vi "Result Set Data.vi"(8 "error in":errorcluster, 9 "Set Data":T1={"UUT_TEST_INFO"={"ID"="", "STATION_ID"="", "TEST_SOCKET_INDEX"="", "UUT_SERIAL_NUMBER"="", "TSW_VER"="", "VAL_SW_VER"="", "PROJECT_NAME"="", "PRODUCT_NAME"="", "PRODUCT_VARIANT"="", "TEST_NAME"="", "TEST_PHASE"="", "TEST_DESCRIPTION"="", "TEMP_CHAMBER_NAME"="", "START_DATE_TIME"="", "STOP_DATE_TIME "="", "START_CYCLE_COUNT"="", "STOP_CYCLE_COUNT"="", "EXECUTION_TIME"="", "UUT_STATUS"="", "UUT_ERROR_CODE"="", "UUT_ERROR_MESSAGE"="", "TEST_SEQUENCE"=""}, "FE_FRAME_LOG"={"ID"="", "UUT_TEST_INFO"="", "DATE_TIME"="", "CYCLE_NUMBER"="", "TEST_MODE"="", "CHAMBER_TEMP"="", "CAN_FRAME_RX"="", "Test Mode"=0, "LV_PPS_VOLTAGE"="", "LV_PPS_CURRENT"="", "HV_PPS_VOLTAGE"="", "HV_PPS_CURRENT"="", "SOCKET_NUMBER"="", "CAN_FRAME_RX_NO_OFF_BYTE"=""}, "FF_FRAME_LOG"={"ID"="", "UUT_TEST_INFO"="", "DATE_TIME"="", "CYCLE_NUMBER"="", "TEST_MODE"="", "CAN_FRAME_RX"="", "CHAMBER_TEMP"="", "TestMode"=0, "SOCKET_NUMBER"="", "CAN_FRAME_RX_NO_OFF_BYTE"=""}, "LIMIT_TABLE"={"ID"="", "PRODUCT_NAME"="", "PRODUCT_VARIANT"="", "TEST_MODE"="", "PARAMETER_NAME"="", "COMPARISON_TYPE"="", "LOW_LIMIT"="", "HIGH_LIMIT"="", "UNIT"="", "ERROR_MESSSAGE"="", "SEVERITY"=""}, "ERROR LOG Append"=[], "FA_FRAME_LOG"={"UUT_TEST_INFO"="", "CAN_FRAME_RX"="", "CAN_FRAME_RX_NO_OFF_BYTE"=""}, "Socket No"=1, "TEST RESULT LOG Append"=[], "SYSTEM_LOG"={"ID "="", "DATE_TIME"="", "CYCLE_NUMBER"="", "TEST_MODE"="", "ERROR_MESSAGE"=""}, "Temperature log"={"TEST_MODE"="", "CYCLE_NUMBER"="", "TEMPERATURE"={"LV_PPS_TEMPERATURE"=0.0, "HV_PPS1_TEMPERATURE"=0.0, "HV_PPS2_TEMPERATURE"=0.0, "HV_PPS3_TEMPERATURE"=0.0, "HV_PPS4_TEMPERATURE"=0.0, "HV_PPS5_TEMPERATURE"=0.0, "HV_PPS6_TEMPERATURE"=0.0, "CHAMBER_TEMPERATURE"=0.0, "LOAD_U1_TEMPERATURE"=0.0, "LOAD_V1_TEMPERATURE"=0.0, "LOAD_W1_TEMPERATURE"=0.0, "LOAD_U2_TEMPERATURE"=0.0, "LOAD_V2_TEMPERATURE"=0.0, "LOAD_W2_TEMPERATURE"=0.0, "LOAD_U3_TEMPERATURE"=0.0, "LOAD_V3_TEMPERATURE"=0.0, "LOAD_W3_TEMPERATURE"=0.0}, "Temperature Inrange"={"LVPPS_Trip?"=FALSE, "HVPPS1_Trip?"=FALSE, "HVPPS2_Trip?"=FALSE, "HVPPS3_Trip?"=FALSE, "HVPPS4_Trip?"=FALSE, "HVPPS5_Trip?"=FALSE, "HVPPS6_Trip?"=FALSE, "Chamber_Trip?"=FALSE}}, "POWER_STATUS"={"TEST_MODE"="", "CYCLE_NUMBER"="", "TYPE_POWER"="", "STATE"=""}, "CYCLE_DURATION_LOG"={"CYCLE_NUMBER"=""}}, 10 "Table Name":string, 11 "Action":enum16{"Insert", "Update"}(ring)) -> (0 "error out":errorcluster)   [LabVIEW 2023, in "HardwareAbstractionLayer_LVOOP.lvlib" / "Report.lvclass"]
uses:
  Report.lvclass
  Control/All Log Details.ctl
  Control/UUT Test Info.ctl
  Control/FE FRAME LOG.ctl
  Control/FF FRAME LOG.ctl
  Control/LIMIT TABLE.ctl
  Control/ERROR LOG APPEND.ctl
  Control/ERROR LOG.ctl
  Control/FA FRAME LOG.ctl
  Control/TEST RESULT LOG APPEND.ctl
  Control/TEST RESULT LOG.ctl
  Control/SYSTEM LOG.ctl
  Control/Temperature LOG.ctl
  Control/POWER STATUS.ctl
  Control/CYCLE_DURATION_LOG.ctl
  Control/Queue FGV.ctl
  Control/Q Data.ctl
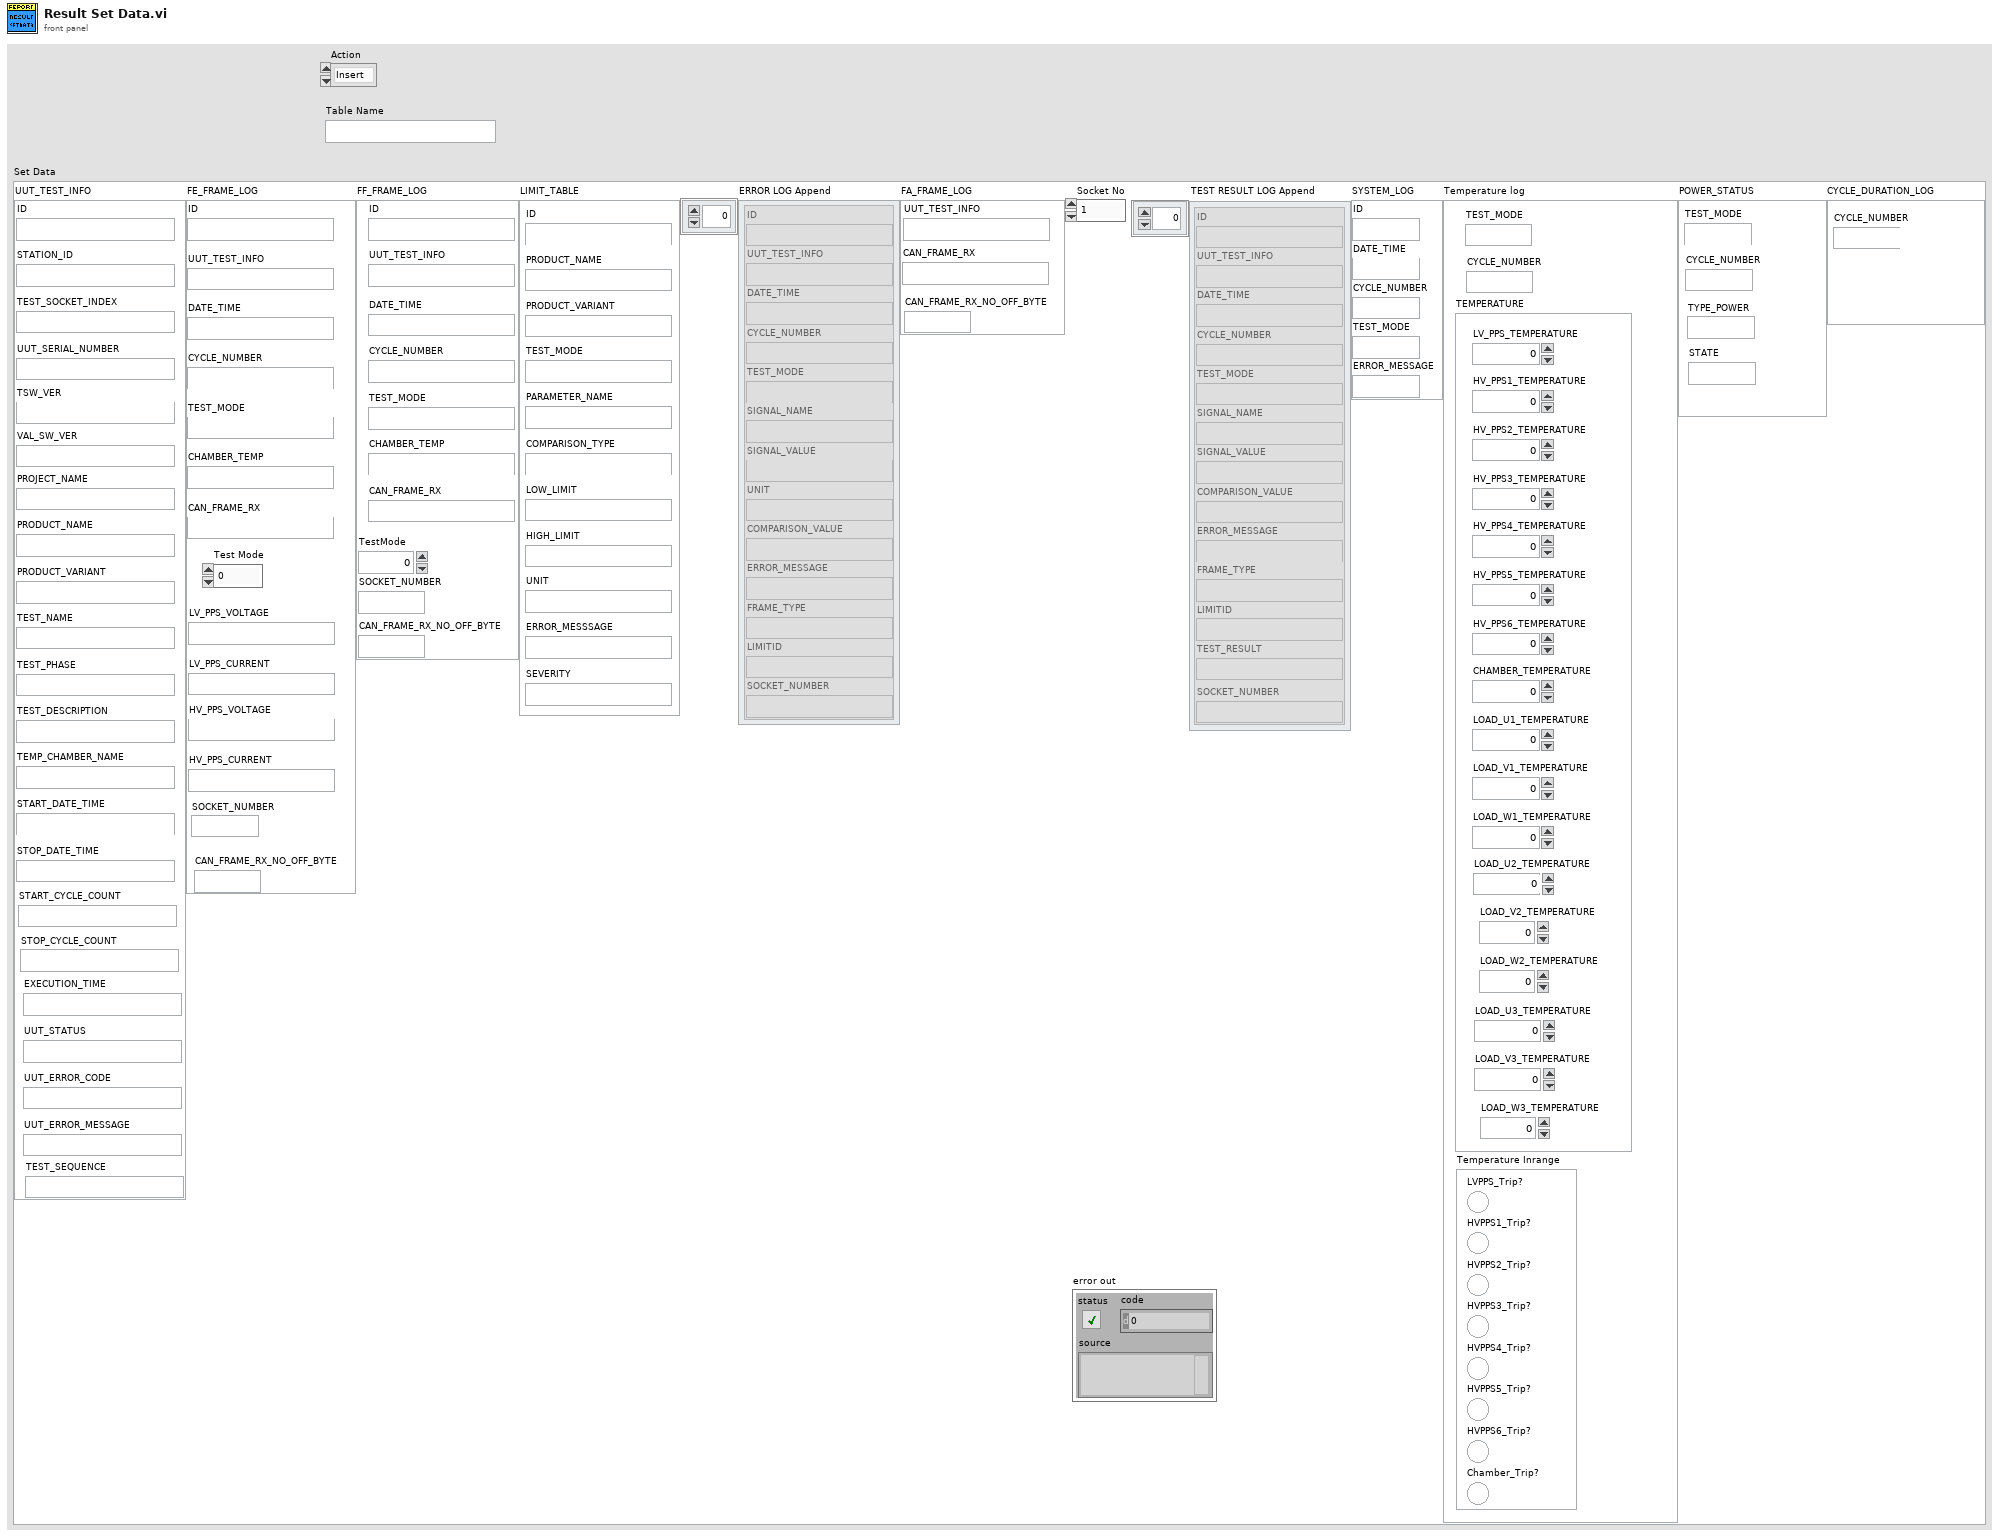
[diagram p1: front panel]
types:
  T1 = typedef "HardwareAbstractionLayer_LVOOP.lvlib/Report.lvclass/All Log Details.ctl" = cluster{"UUT_TEST_INFO":T2, "FE_FRAME_LOG":T3, "FF_FRAME_LOG":T4, "LIMIT_TABLE":T5, "ERROR LOG Append":T6, "FA_FRAME_LOG":T8, "Socket No":u16, "TEST RESULT LOG Append":T9, "SYSTEM_LOG":T11, "Temperature log":T12, "POWER_STATUS":T13, "CYCLE_DURATION_LOG":T14}
  T2 = typedef "HardwareAbstractionLayer_LVOOP.lvlib/Report.lvclass/UUT Test Info.ctl" = cluster{"ID":string, "STATION_ID":string, "TEST_SOCKET_INDEX":string, "UUT_SERIAL_NUMBER":string, "TSW_VER":string, "VAL_SW_VER":string, "PROJECT_NAME":string, "PRODUCT_NAME":string, "PRODUCT_VARIANT":string, "TEST_NAME":string, "TEST_PHASE":string, "TEST_DESCRIPTION":string, "TEMP_CHAMBER_NAME":string, "START_DATE_TIME":string, "STOP_DATE_TIME ":string, "START_CYCLE_COUNT":string, "STOP_CYCLE_COUNT":string, "EXECUTION_TIME":string, "UUT_STATUS":string, "UUT_ERROR_CODE":string, "UUT_ERROR_MESSAGE":string, "TEST_SEQUENCE":string}
  T3 = typedef "HardwareAbstractionLayer_LVOOP.lvlib/Report.lvclass/FE FRAME LOG.ctl" = cluster{"ID":string, "UUT_TEST_INFO":string, "DATE_TIME":string, "CYCLE_NUMBER":string, "TEST_MODE":string, "CHAMBER_TEMP":string, "CAN_FRAME_RX":string, "Test Mode":u32, "LV_PPS_VOLTAGE":string, "LV_PPS_CURRENT":string, "HV_PPS_VOLTAGE":string, "HV_PPS_CURRENT":string, "SOCKET_NUMBER":string, "CAN_FRAME_RX_NO_OFF_BYTE":string}
  T4 = typedef "HardwareAbstractionLayer_LVOOP.lvlib/Report.lvclass/FF FRAME LOG.ctl" = cluster{"ID":string, "UUT_TEST_INFO":string, "DATE_TIME":string, "CYCLE_NUMBER":string, "TEST_MODE":string, "CAN_FRAME_RX":string, "CHAMBER_TEMP":string, "TestMode":u32, "SOCKET_NUMBER":string, "CAN_FRAME_RX_NO_OFF_BYTE":string}
  T5 = typedef "HardwareAbstractionLayer_LVOOP.lvlib/Report.lvclass/LIMIT TABLE.ctl" = cluster{"ID":string, "PRODUCT_NAME":string, "PRODUCT_VARIANT":string, "TEST_MODE":string, "PARAMETER_NAME":string, "COMPARISON_TYPE":string, "LOW_LIMIT":string, "HIGH_LIMIT":string, "UNIT":string, "ERROR_MESSSAGE":string, "SEVERITY":string}
  T6 = typedef "HardwareAbstractionLayer_LVOOP.lvlib/Report.lvclass/ERROR LOG APPEND.ctl" = T7[]
  T7 = typedef "HardwareAbstractionLayer_LVOOP.lvlib/Report.lvclass/ERROR LOG.ctl" = cluster{"ID":string, "UUT_TEST_INFO":string, "DATE_TIME":string, "CYCLE_NUMBER":string, "TEST_MODE":string, "SIGNAL_NAME":string, "SIGNAL_VALUE":string, "UNIT":string, "COMPARISON_VALUE":string, "ERROR_MESSAGE":string, "FRAME_TYPE":string, "LIMITID":string, "SOCKET_NUMBER":string}
  T8 = typedef "HardwareAbstractionLayer_LVOOP.lvlib/Report.lvclass/FA FRAME LOG.ctl" = cluster{"UUT_TEST_INFO":string, "CAN_FRAME_RX":string, "CAN_FRAME_RX_NO_OFF_BYTE":string}
  T9 = typedef "HardwareAbstractionLayer_LVOOP.lvlib/Report.lvclass/TEST RESULT LOG APPEND.ctl" = T10[]
  T10 = typedef "HardwareAbstractionLayer_LVOOP.lvlib/Report.lvclass/TEST RESULT LOG.ctl" = cluster{"ID":string, "UUT_TEST_INFO":string, "DATE_TIME":string, "CYCLE_NUMBER":string, "TEST_MODE":string, "SIGNAL_NAME":string, "SIGNAL_VALUE":string, "COMPARISON_VALUE":string, "ERROR_MESSAGE":string, "FRAME_TYPE":string, "LIMITID":string, "TEST_RESULT":string, "SOCKET_NUMBER":string}
  T11 = typedef "HardwareAbstractionLayer_LVOOP.lvlib/Report.lvclass/SYSTEM LOG.ctl" = cluster{"ID ":string, "DATE_TIME":string, "CYCLE_NUMBER":string, "TEST_MODE":string, "ERROR_MESSAGE":string}
  T12 = typedef "HardwareAbstractionLayer_LVOOP.lvlib/Report.lvclass/Temperature LOG.ctl" = cluster{"TEST_MODE":string, "CYCLE_NUMBER":string, "TEMPERATURE":cluster{"LV_PPS_TEMPERATURE":dbl, "HV_PPS1_TEMPERATURE":dbl, "HV_PPS2_TEMPERATURE":dbl, "HV_PPS3_TEMPERATURE":dbl, "HV_PPS4_TEMPERATURE":dbl, "HV_PPS5_TEMPERATURE":dbl, "HV_PPS6_TEMPERATURE":dbl, "CHAMBER_TEMPERATURE":dbl, "LOAD_U1_TEMPERATURE":dbl, "LOAD_V1_TEMPERATURE":dbl, "LOAD_W1_TEMPERATURE":dbl, "LOAD_U2_TEMPERATURE":dbl, "LOAD_V2_TEMPERATURE":dbl, "LOAD_W2_TEMPERATURE":dbl, "LOAD_U3_TEMPERATURE":dbl, "LOAD_V3_TEMPERATURE":dbl, "LOAD_W3_TEMPERATURE":dbl}, "Temperature Inrange":cluster{"LVPPS_Trip?":bool, "HVPPS1_Trip?":bool, "HVPPS2_Trip?":bool, "HVPPS3_Trip?":bool, "HVPPS4_Trip?":bool, "HVPPS5_Trip?":bool, "HVPPS6_Trip?":bool, "Chamber_Trip?":bool}}
  T13 = typedef "HardwareAbstractionLayer_LVOOP.lvlib/Report.lvclass/POWER STATUS.ctl" = cluster{"TEST_MODE":string, "CYCLE_NUMBER":string, "TYPE_POWER":string, "STATE":string}
  T14 = typedef "HardwareAbstractionLayer_LVOOP.lvlib/Report.lvclass/CYCLE_DURATION_LOG.ctl" = cluster{"CYCLE_NUMBER":string}
  T15 = typedef "HardwareAbstractionLayer_LVOOP.lvlib/Report.lvclass/Q Data.ctl" = cluster{"Table Name":string, "Data":variant, "Action":enum16{"Insert", "Update"}, "Schema":string, "Socket No":u16}
  T16 = typedef "HardwareAbstractionLayer_LVOOP.lvlib/Report.lvclass/Queue FGV.ctl" = enum16{"Init", "Set", "Get"}
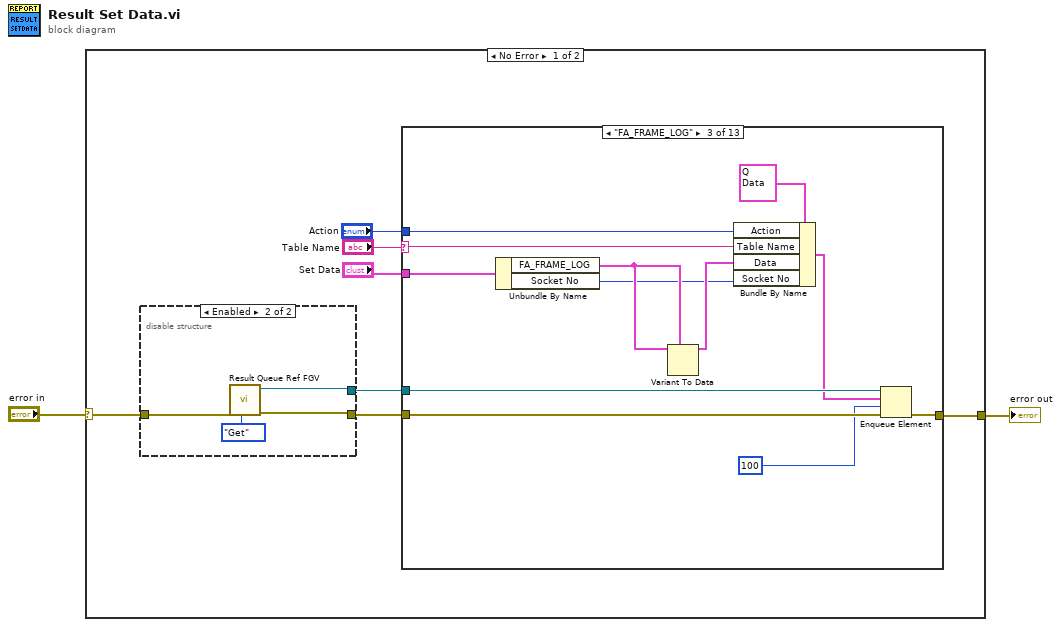
[diagram p0: block diagram]
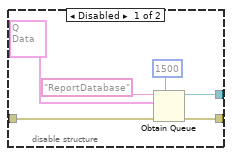
[diagram p2: hidden frame]
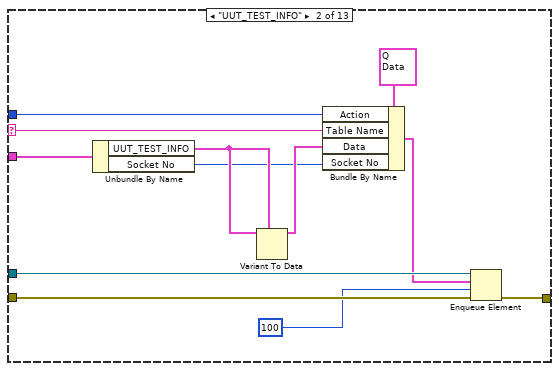
[diagram p4: hidden frame]
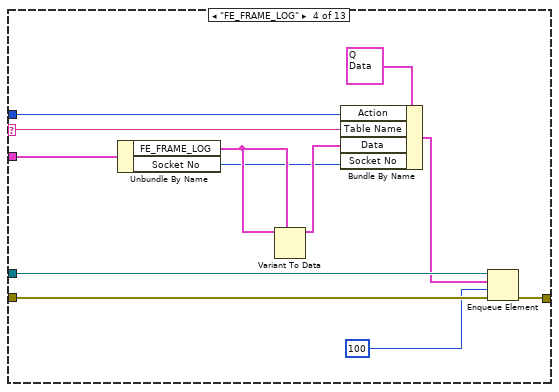
[diagram p5: hidden frame]
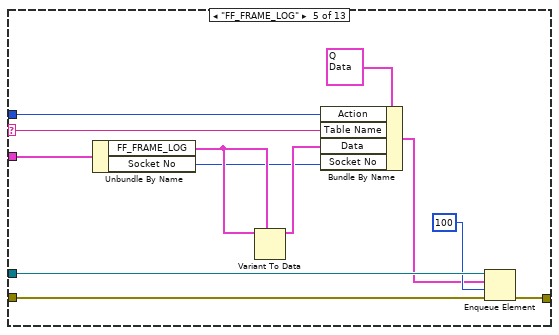
[diagram p6: hidden frame]
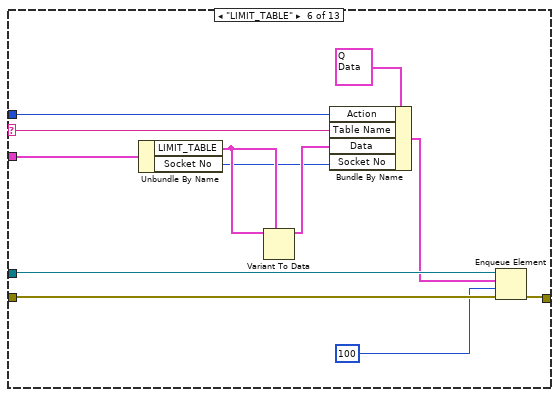
[diagram p7: hidden frame]
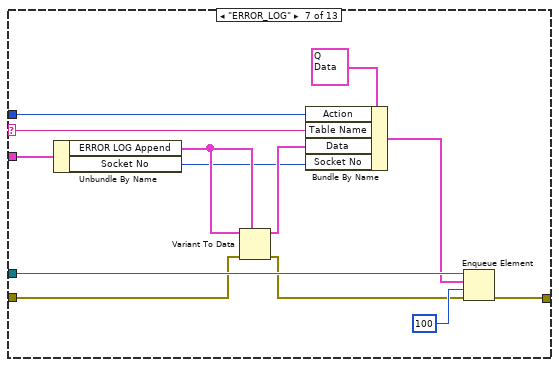
[diagram p8: hidden frame]
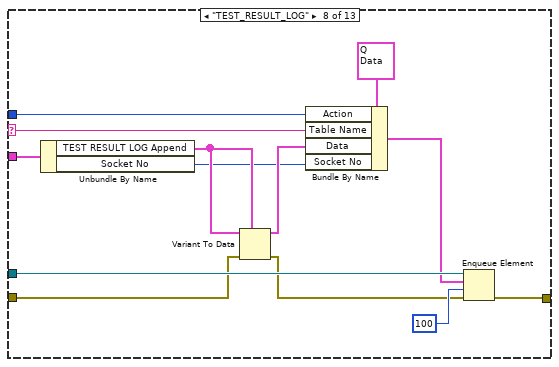
[diagram p9: hidden frame]
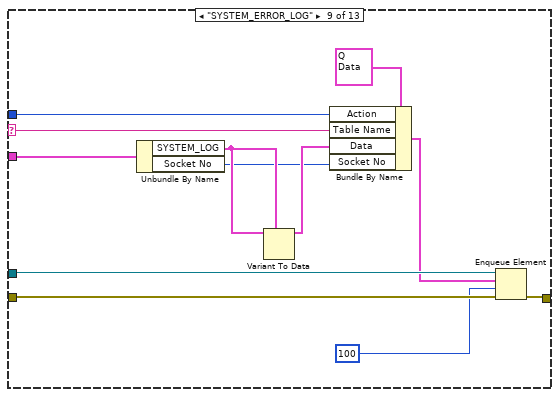
[diagram p10: hidden frame]
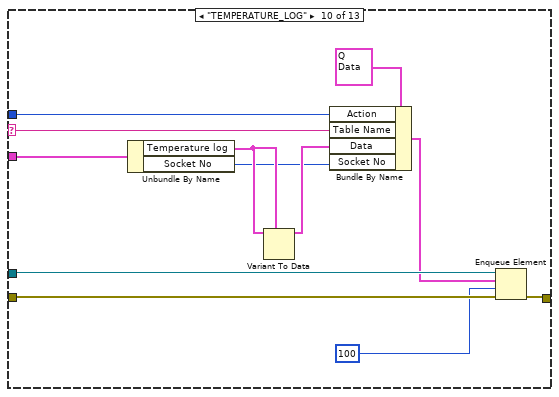
[diagram p11: hidden frame]
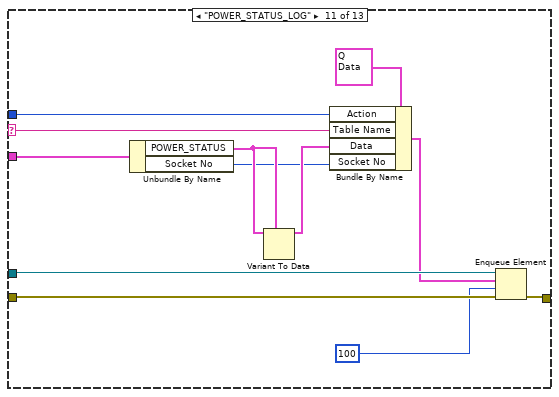
[diagram p12: hidden frame]
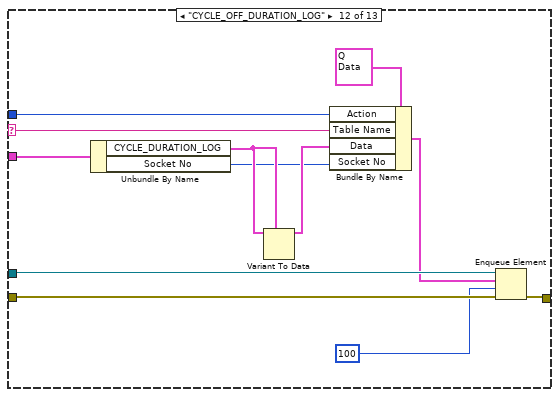
[diagram p13: hidden frame]
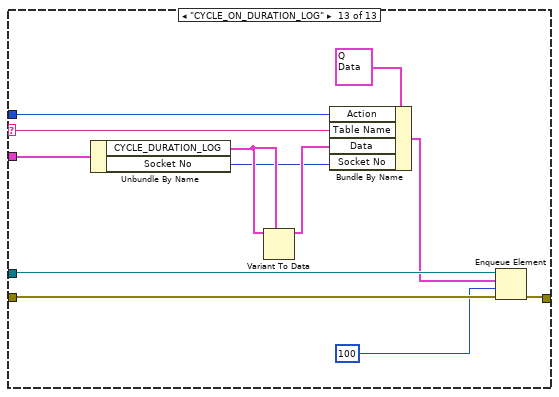
[diagram p14: hidden frame]
diagram:
  n1 = case shown="No Error" "error in" {
    selector: "error in" -> [w3 w167]
    tunnel: [w4 w167] -> w1
    frame No Error {
      n2 = disable-structure shown="Enabled" {
        disable-tunnel: [w12 w16] -> w9
        disable-tunnel: [w11 w18] -> w8
        disable-tunnel: w3 -> [w10 w19]
        frame Disabled {
          n3 = Obtain Queue(max queue size (-1, unlimited)=1500, name (unnamed)="ReportDatabase", element data type=T15 {"Table Name"="", "Data"=variant, "Action"=enum."Insert", "Schema"="", "Socket No"=1} ("Q Data"), error in (no error)=w10) -> (queue out=w12:refnum<queue>, error out=w11:errorcluster)  [unwired: 1 in, 1 out]
        }
        frame Enabled {
          n4 = call "Result Queue Ref FGV.vi"("Q FGV"=Queue_FGV."Get", "error in"=w19) -> ("error out"=w18:errorcluster, "Get Queue"=w16:refnum<queue>)  [unwired: 8 in]
        }
      }
      n5 = case shown="\"FA_FRAME_LOG\"" "Table Name" {
        selector: "Table Name" -> [_ w25 w38 w50 w61 w73 w89 w102 w111 w123 w135 w147 w159]
        tunnel: w9 -> [_ w32 w44 w56 w68 w80 w93 w106 w118 w130 w142 w154 w166]
        tunnel: w8 -> [w20 w31 w43 w55 w67 w79 w86 w99 w117 w129 w141 w153 w165]
        tunnel: "Set Data" -> [_ w24 w39 w51 w62 w72 w91 w104 w110 w122 w134 w146 w158]
        tunnel: "Action" -> [_ w26 w37 w49 w60 w74 w83 w96 w112 w124 w136 w148 w160]
        tunnel: [w20 w22 w34 w46 w58 w70 w82 w95 w108 w120 w132 w144 w156] -> w4
        frame "False", Default {
        }
        frame "UUT_TEST_INFO" {
          n6 = Unbundle By Name(w24) -> ("UUT_TEST_INFO"=w27:T2, "Socket No"=w21:u16)
          n7 = Variant To Data(type=w27, Variant=w27) -> (data=w28:T2)  [unwired: 1 in, 1 out]
          n8 = Bundle By Name(cluster=T15 {"Table Name"="", "Data"=variant, "Action"=enum."Insert", "Schema"="", "Socket No"=1} ("element"), "Action"=w26, "Table Name"=w25, "Data"=w28, "Socket No"=w21) -> (w23:T15)
          n9 = Enqueue Element(queue=w32, element=w23, timeout in ms (-1)=100, error in (no error)=w31) -> (error out=w22:errorcluster)  [unwired: 2 out]
        }
        frame "FA_FRAME_LOG" {
          n10 = Unbundle By Name(w39) -> ("FA_FRAME_LOG"=w40:T8, "Socket No"=w33:u16)
          n11 = Variant To Data(type=w40, Variant=w40) -> (data=w41:T8)  [unwired: 1 in, 1 out]
          n12 = Bundle By Name(cluster=T15 {"Table Name"="", "Data"=variant, "Action"=enum."Insert", "Schema"="", "Socket No"=1} ("element"), "Action"=w37, "Table Name"=w38, "Data"=w41, "Socket No"=w33) -> (w35:T15)
          n13 = Enqueue Element(queue=w44, element=w35, timeout in ms (-1)=100, error in (no error)=w43) -> (error out=w34:errorcluster)  [unwired: 2 out]
        }
        frame "FE_FRAME_LOG" {
          n14 = Unbundle By Name(w51) -> ("FE_FRAME_LOG"=w52:T3, "Socket No"=w45:u16)
          n15 = Variant To Data(type=w52, Variant=w52) -> (data=w53:T3)  [unwired: 1 in, 1 out]
          n16 = Bundle By Name(cluster=T15 {"Table Name"="", "Data"=variant, "Action"=enum."Insert", "Schema"="", "Socket No"=1} ("element"), "Action"=w49, "Table Name"=w50, "Data"=w53, "Socket No"=w45) -> (w47:T15)
          n17 = Enqueue Element(queue=w56, element=w47, timeout in ms (-1)=100, error in (no error)=w55) -> (error out=w46:errorcluster)  [unwired: 2 out]
        }
        frame "FF_FRAME_LOG" {
          n18 = Unbundle By Name(w62) -> ("FF_FRAME_LOG"=w63:T4, "Socket No"=w57:u16)
          n19 = Variant To Data(type=w63, Variant=w63) -> (data=w64:T4)  [unwired: 1 in, 1 out]
          n20 = Bundle By Name(cluster=T15 {"Table Name"="", "Data"=variant, "Action"=enum."Insert", "Schema"="", "Socket No"=1} ("element"), "Action"=w60, "Table Name"=w61, "Data"=w64, "Socket No"=w57) -> (w59:T15)
          n21 = Enqueue Element(queue=w68, element=w59, timeout in ms (-1)=100, error in (no error)=w67) -> (error out=w58:errorcluster)  [unwired: 2 out]
        }
        frame "LIMIT_TABLE" {
          n22 = Unbundle By Name(w72) -> ("LIMIT_TABLE"=w75:T5, "Socket No"=w69:u16)
          n23 = Variant To Data(type=w75, Variant=w75) -> (data=w76:T5)  [unwired: 1 in, 1 out]
          n24 = Bundle By Name(cluster=T15 {"Table Name"="", "Data"=variant, "Action"=enum."Insert", "Schema"="", "Socket No"=1} ("element"), "Action"=w74, "Table Name"=w73, "Data"=w76, "Socket No"=w69) -> (w71:T15)
          n25 = Enqueue Element(queue=w80, element=w71, timeout in ms (-1)=100, error in (no error)=w79) -> (error out=w70:errorcluster)  [unwired: 2 out]
        }
        frame "ERROR_LOG" {
          n26 = Unbundle By Name(w91) -> ("ERROR LOG Append"=w84:T6, "Socket No"=w81:u16)
          n27 = Variant To Data(error in=w86, type=w84, Variant=w84) -> (data=w87:T6, error out=w85:errorcluster)
          n28 = Bundle By Name(cluster=T15 {"Table Name"="", "Data"=variant, "Action"=enum."Insert", "Schema"="", "Socket No"=1} ("element"), "Action"=w83, "Table Name"=w89, "Data"=w87, "Socket No"=w81) -> (w88:T15)
          n29 = Enqueue Element(queue=w93, element=w88, timeout in ms (-1)=100, error in (no error)=w85) -> (error out=w82:errorcluster)  [unwired: 2 out]
        }
        frame "TEST_RESULT_LOG" {
          n30 = Unbundle By Name(w104) -> ("TEST RESULT LOG Append"=w97:T9, "Socket No"=w94:u16)
          n31 = Variant To Data(error in=w99, type=w97, Variant=w97) -> (data=w100:T9, error out=w98:errorcluster)
          n32 = Bundle By Name(cluster=T15 {"Table Name"="", "Data"=variant, "Action"=enum."Insert", "Schema"="", "Socket No"=1} ("element"), "Action"=w96, "Table Name"=w102, "Data"=w100, "Socket No"=w94) -> (w101:T15)
          n33 = Enqueue Element(queue=w106, element=w101, timeout in ms (-1)=100, error in (no error)=w98) -> (error out=w95:errorcluster)  [unwired: 2 out]
        }
        frame "SYSTEM_ERROR_LOG" {
          n34 = Unbundle By Name(w110) -> ("SYSTEM_LOG"=w113:T11, "Socket No"=w107:u16)
          n35 = Variant To Data(type=w113, Variant=w113) -> (data=w114:T11)  [unwired: 1 in, 1 out]
          n36 = Bundle By Name(cluster=T15 {"Table Name"="", "Data"=variant, "Action"=enum."Insert", "Schema"="", "Socket No"=1} ("element"), "Action"=w112, "Table Name"=w111, "Data"=w114, "Socket No"=w107) -> (w109:T15)
          n37 = Enqueue Element(queue=w118, element=w109, timeout in ms (-1)=100, error in (no error)=w117) -> (error out=w108:errorcluster)  [unwired: 2 out]
        }
        frame "TEMPERATURE_LOG" {
          n38 = Unbundle By Name(w122) -> ("Temperature log"=w125:T12, "Socket No"=w119:u16)
          n39 = Variant To Data(type=w125, Variant=w125) -> (data=w126:T12)  [unwired: 1 in, 1 out]
          n40 = Bundle By Name(cluster=T15 {"Table Name"="", "Data"=variant, "Action"=enum."Insert", "Schema"="", "Socket No"=1} ("element"), "Action"=w124, "Table Name"=w123, "Data"=w126, "Socket No"=w119) -> (w121:T15)
          n41 = Enqueue Element(queue=w130, element=w121, timeout in ms (-1)=100, error in (no error)=w129) -> (error out=w120:errorcluster)  [unwired: 2 out]
        }
        frame "POWER_STATUS_LOG" {
          n42 = Unbundle By Name(w134) -> ("POWER_STATUS"=w137:T13, "Socket No"=w131:u16)
          n43 = Variant To Data(type=w137, Variant=w137) -> (data=w138:T13)  [unwired: 1 in, 1 out]
          n44 = Bundle By Name(cluster=T15 {"Table Name"="", "Data"=variant, "Action"=enum."Insert", "Schema"="", "Socket No"=1} ("element"), "Action"=w136, "Table Name"=w135, "Data"=w138, "Socket No"=w131) -> (w133:T15)
          n45 = Enqueue Element(queue=w142, element=w133, timeout in ms (-1)=100, error in (no error)=w141) -> (error out=w132:errorcluster)  [unwired: 2 out]
        }
        frame "CYCLE_OFF_DURATION_LOG" {
          n46 = Unbundle By Name(w146) -> ("CYCLE_DURATION_LOG"=w149:T14, "Socket No"=w143:u16)
          n47 = Variant To Data(type=w149, Variant=w149) -> (data=w150:T14)  [unwired: 1 in, 1 out]
          n48 = Bundle By Name(cluster=T15 {"Table Name"="", "Data"=variant, "Action"=enum."Insert", "Schema"="", "Socket No"=1} ("element"), "Action"=w148, "Table Name"=w147, "Data"=w150, "Socket No"=w143) -> (w145:T15)
          n49 = Enqueue Element(queue=w154, element=w145, timeout in ms (-1)=100, error in (no error)=w153) -> (error out=w144:errorcluster)  [unwired: 2 out]
        }
        frame "CYCLE_ON_DURATION_LOG" {
          n50 = Unbundle By Name(w158) -> ("CYCLE_DURATION_LOG"=w161:T14, "Socket No"=w155:u16)
          n51 = Variant To Data(type=w161, Variant=w161) -> (data=w162:T14)  [unwired: 1 in, 1 out]
          n52 = Bundle By Name(cluster=T15 {"Table Name"="", "Data"=variant, "Action"=enum."Insert", "Schema"="", "Socket No"=1} ("element"), "Action"=w160, "Table Name"=w159, "Data"=w162, "Socket No"=w155) -> (w157:T15)
          n53 = Enqueue Element(queue=w166, element=w157, timeout in ms (-1)=100, error in (no error)=w165) -> (error out=w156:errorcluster)  [unwired: 2 out]
        }
      }
    }
    frame Error {
    }
  }
  "error out" <- w1
